vi "Line ROI to Pixels.vi"(8 "error in (no error)":errorcluster, 11 "ROI":T1) -> (0 "error out":errorcluster, 3 "pixel dist":dbl)   [LabVIEW 2020]
uses:
  <vilib>/vision/NI_Vision_Development_Module.lvlib
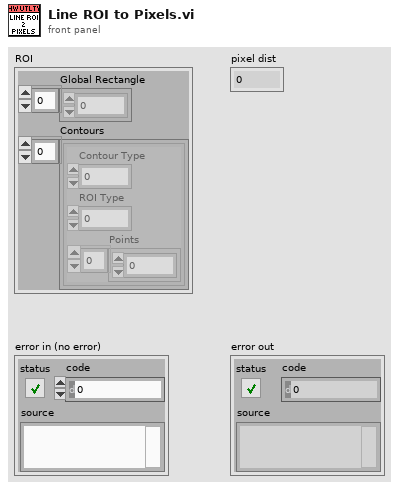
[diagram p1: front panel]
types:
  T1 = cluster{"Global Rectangle":i32[], "Contours":cluster{"Contour Type":u32, "ROI Type":u32, "Points":i32[]}[]}
  T2 = cluster{"Contour Type":u32, "ROI Type":u32, "Points":i32[]}[]
  T3 = cluster{"Contour Type":u32, "ROI Type":u32, "Points":i32[]}
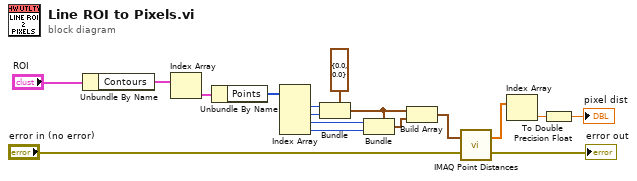
[diagram p0: block diagram]
diagram:
  n1 = Unbundle By Name("ROI") -> ("Contours"=w14:T2)
  n2 = Index Array(array=w14) -> (element=w15:T3)  [unwired: 1 in]
  n3 = Unbundle By Name(w15) -> ("Points"=w16:i32[])
  n4 = Index Array(array=w16) -> (element #1=w2:i32, element #2=w3:i32, element #3=w5:i32, element #4=w6:i32)  [unwired: 4 in]
  n5 = Bundle(cluster=cluster{"X":sgl, "Y":sgl} {"X"=0.0, "Y"=0.0}, "X"=w2, "Y"=w3) -> (w7:cluster{"X":sgl, "Y":sgl})
  n6 = Bundle(cluster=w7, "X"=w5, "Y"=w6) -> (w8:cluster{"X":sgl, "Y":sgl})
  n7 = Build Array(w7, w8) -> (w9:cluster{"X":sgl, "Y":sgl}[])
  n8 = call "IMAQ Point Distances"("Points"=w9, "error in (no error)"="error in (no error)") -> ("Distances"=w10:sgl[], "error out"=→"error out":errorcluster)  [unwired: 3 in]
  n9 = Index Array(array=w10) -> (element=w11:sgl)  [unwired: 1 in]
  n10 = To Double Precision Float(number=w11) -> (double precision float=→"pixel dist":dbl)
